vi "get ext error.vi"(5 "connection reference":T1, 6 "length":i32=1, 7 "sample data list":T2, 9 "seq std":dbl[][](array[numeric]), 10 "sample data":string[][](array[string]), 11 "unknown data in":dbl[][][](array[numeric])) -> (2 "normalized ratio":dbl[](array[numeric]), 3 "Array out":string[][](array[string]))   [LabVIEW 2016]
uses:
  <vilib>/addons/database/Connection.llb/Conn ObjectReference.ctl
  <vilib>/Analysis/baseanly.llb/Mean (DBL).vi
  <vilib>/addons/database/Connection.llb/Conn Execute.vi
  <vilib>/addons/database/Recordset.llb/Rec Fetch Recordset Data (R).vi
  <vilib>/addons/database/Recordset.llb/Rec Destroy - Connection.vi
  <vilib>/addons/database/NI_Database_API.lvlib
  <vilib>/Analysis/NI_AALBase.lvlib
panel:
  out "error out":errorcluster
  out "Array 2":string[][](array[string])
  out "unknown data in 4":dbl[][](array[numeric])
  out "subarray":dbl[](array[numeric])
  out "unknown data in 3":dbl[][](array[numeric])
  out "unknown data in 2":dbl[](array[numeric])
  out "Array":dbl[](array[numeric])
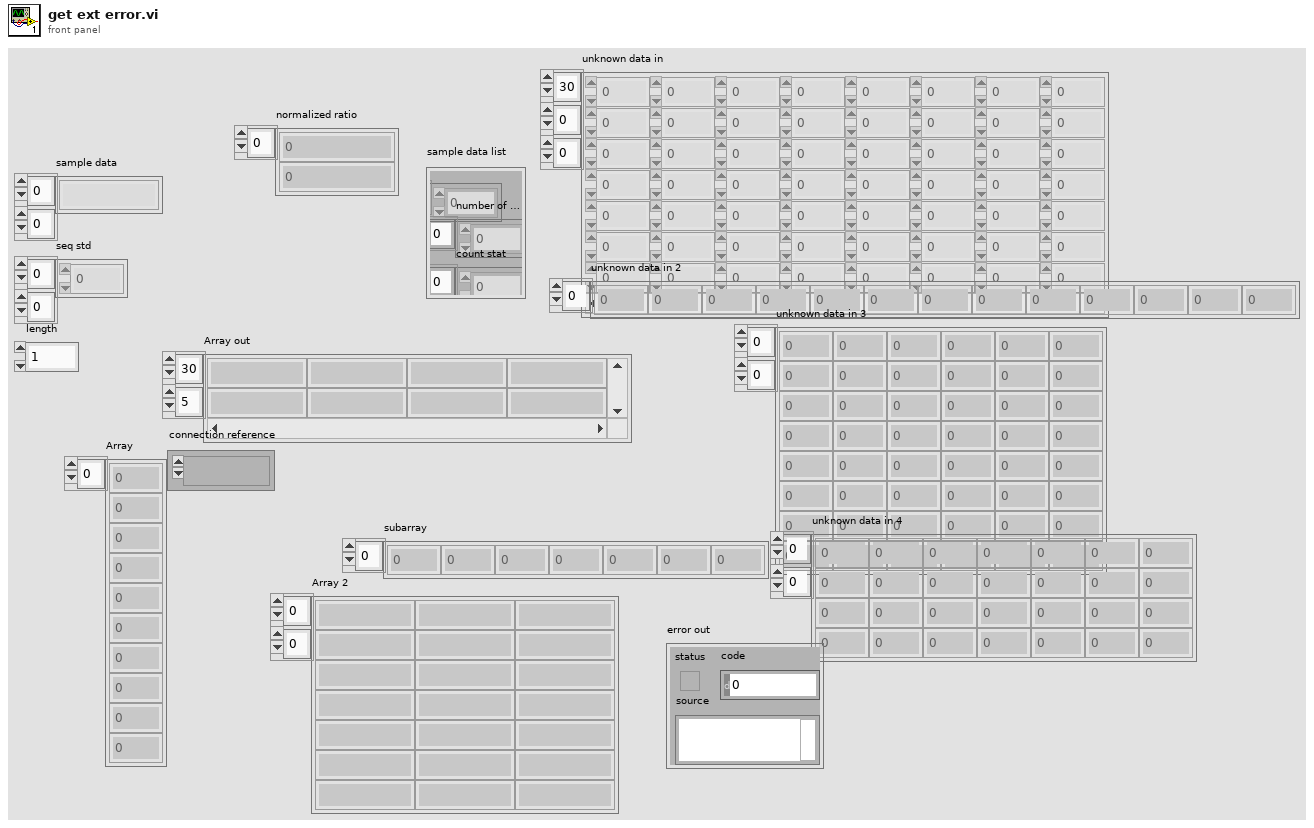
[diagram p1: front panel]
types:
  T1 = typedef "NI_Database_API.lvlib/Conn ObjectReference.ctl" = refnum<k1>
  T2 = cluster{"last currents":dbl[], "number of cycles":i32[], "count stat":dbl[]}
  T3 = typedef "NI_Database_API.lvlib/Rec ObjectReference.ctl" = refnum<k1>
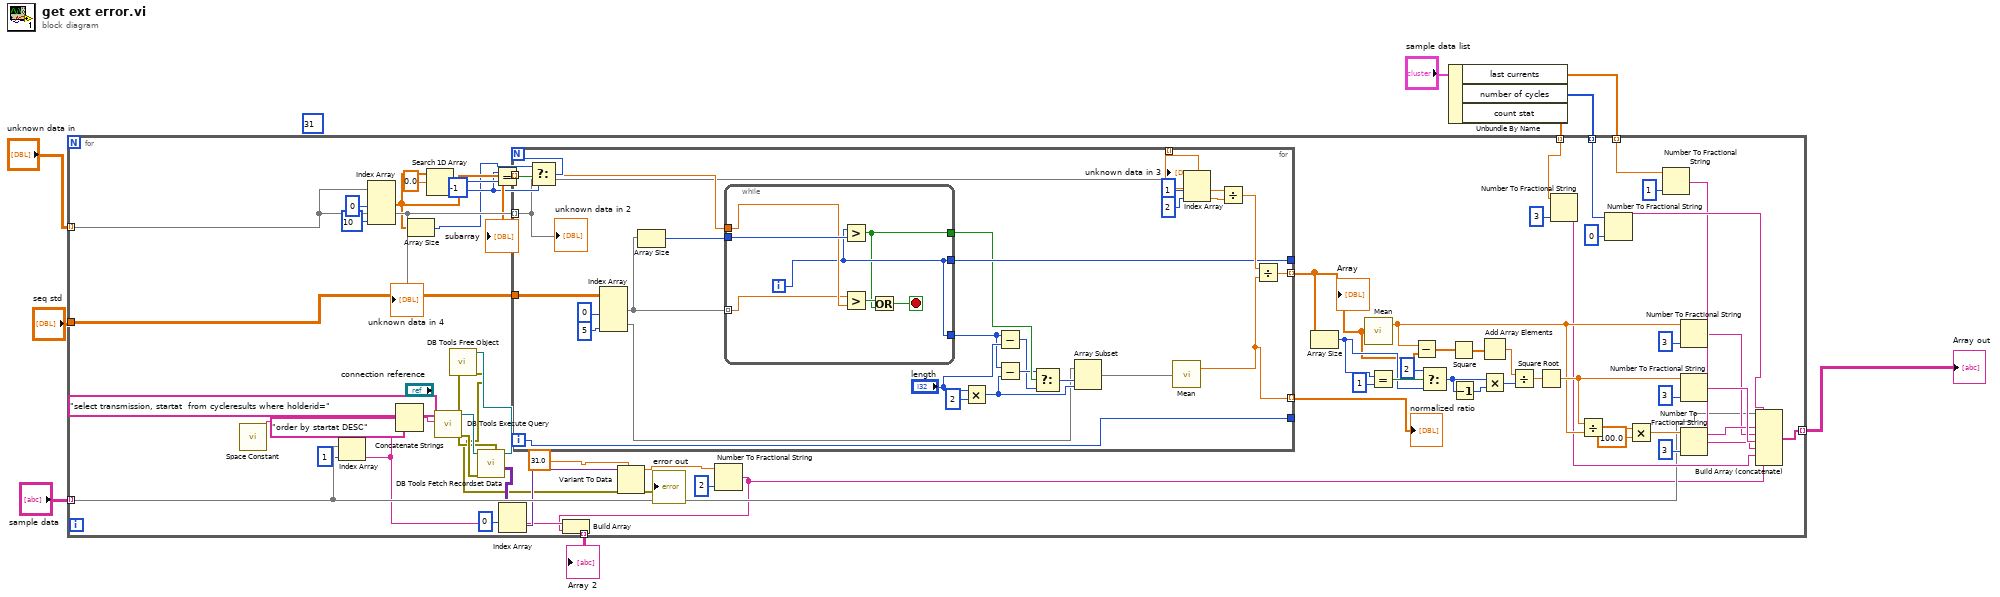
[diagram p0: block diagram]
diagram:
  (unwired) 31
  n1 = Unbundle By Name("sample data list") -> ("last currents"=w3:dbl[], "number of cycles"=w5:i32[], "count stat"=w4:dbl[])
  n2 = for {
    tunnel: "unknown data in" -> [w72] mode=indexing
    tunnel: "seq std" -> [w76]
    tunnel: "sample data" -> [w26] mode=indexing
    tunnel: [w74] -> w2 mode=indexing
    tunnel: w5 -> [w42] mode=indexing
    tunnel: w4 -> [w39] mode=indexing
    tunnel: w3 -> [w37] mode=indexing
    tunnel: [w18] -> w1 mode=indexing
    w22 = 0 ("disabled index (col)")
    n3 = call <vilib>:"Space Constant.vi"() -> ("String"=w24:string)
    n4 = Index Array(array=w26, index=1) -> (element=w19:string)
    n5 = Index Array(array=w72, index (col) #1=0 ("disabled index (col)"), index (col) #2=10 ("index (col)")) -> (element #1=w51:dbl[])  [unwired: 2 in, 1 out]
    "subarray" <- w51
    n6 = Concatenate Strings("select transmission, startat  from cycleresults where holderid=" ("string"), w19, w24, "order by startat DESC" ("string")) -> (w28:string)
    n7 = Array Size(array=w51) -> (size(s)=w44:i32)
    n8 = Search 1D Array(1D array=w51, element=0.0) -> (index of element=w48:i32)  [unwired: 1 in]
    n9 = call-poly <vilib>:"DB Tools Execute Query.vi"("SQL query"=w28, "connection reference"="connection reference") -> ("error out"=w30:errorcluster, "recordset reference"=w29:T3)  [unwired: 6 in]
    n10 = call-poly <vilib>:"DB Tools Fetch Recordset Data.vi"("error in (no error)"=w30, "recordset reference"=w29) -> ("error out"=w17:errorcluster, "recordset data"=w23:variant[][], "recordset reference out"=w15:T3)  [unwired: 3 in]
    n11 = call-poly <vilib>:"DB Tools Free Object.vi"("error in (no error)"=w17, "recordset reference"=w15) -> ("error out"=w14:errorcluster)  [unwired: 8 in, 1 out]
    n12 = Equal?(x=w48, y=-1) -> (x = y?=w49:bool)
    n13 = Index Array(array=w23, index (row)=w22, index (col)=w22) -> (element=w21:variant)
    n14 = Select(t=w44, s=w49, f=w48) -> (s? t:f=w33:i32)
    n15 = for {
      N: w33 -> [_]
      tunnel: w76 -> [w99]
      tunnel: w72 -> [w81] mode=indexing
      tunnel: w51 -> [w102] mode=indexing
      tunnel: [w91] -> w47 mode=indexing
      tunnel: [w90] -> _
      tunnel: [w83] -> w46 mode=indexing
      tunnel: [w82] -> _
      tunnel: [w81] -> w32 mode=indexing
      i -> [w82]
      n16 = Index Array(array=w99, index (col) #1=0 ("disabled index (col)"), index (col) #2=5 ("index (col)")) -> (element #1=w101:dbl[], element #2=w78:dbl[])  [unwired: 2 in]
      n17 = Array Size(array=w101) -> (size(s)=w100:i32)
      n18 = while {
        tunnel: w102 -> [w107]
        tunnel: w101 -> [w106] mode=indexing
        tunnel: w100 -> [w108]
        tunnel: [w105] -> w80
        tunnel: [w105] -> w90
        tunnel: [w104] -> w88
        i -> [w105]
        stop <- w109 stop-if-true
        n19 = Greater?(x=w105, y=w108) -> (0:w104:bool)
        n20 = Greater?(x=w106, y=w107) -> (0:w110:bool)
        n21 = Or(x=w110, y=w104) -> (x .or. y?=w109:bool)
      }
      n22 = Multiply(x="length", y=2) -> (x*y=w79:i32)
      n23 = Subtract(x=w80, y="length") -> (x-y=w84:i32)
      n24 = Subtract(x=w80, y=w79) -> (x-y=w86:i32)
      n25 = Select(t=w86, s=w88, f=w84) -> (s? t:f=w85:i32)
      n26 = Array Subset(array=w78, index=w85, length=w79) -> (w89:dbl[])
      n27 = call-poly <vilib>:"Mean.vi"("X"=w89) -> ("mean"=w83:dbl)  [unwired: 1 out]
      n28 = Index Array(array=w81, index #1=1 ("index"), index #2=2 ("index")) -> (element #1=w93:dbl, element #2=w94:dbl)
      n29 = Divide(x=w93, y=w94) -> (x/y=w92:dbl)
      n30 = Divide(x=w92, y=w83) -> (x/y=w91:dbl)
      "unknown data in 2" <- w81
    }
    "normalized ratio" <- w46
    "Array" <- w47
    "unknown data in 3" <- w32
    n31 = Variant To Data(error in=w14, type=31.0, Variant=w21) -> (data=w12:dbl, error out=→"error out":errorcluster)
    n32 = Number To Fractional String(number=w12, precision (6)=i16 2) -> (F-format string=w10:string)  [unwired: 2 in]
    n33 = Build Array(w19, w10) -> (w18:string[])
    n34 = Array Size(array=w47) -> (size(s)=w67:i32)
    n35 = call-poly <vilib>:"Mean.vi"("X"=w47) -> ("mean"=w61:dbl)  [unwired: 1 out]
    n36 = Equal?(x=w67, y=1) -> (x = y?=w69:bool)
    n37 = Subtract(x=w61, y=w47) -> (x-y=w71:dbl[])
    n38 = Select(t=2, s=w69, f=w67) -> (s? t:f=w59:i32)
    n39 = Square(x=w71) -> (x^2=w70:dbl[])
    n40 = Decrement(x=w59) -> (x-1=w58:i32)
    n41 = Add Array Elements(numeric array=w70) -> (sum=w65:dbl)
    n42 = Multiply(x=w59, y=w58) -> (x*y=w57:i32)
    n43 = Divide(x=w65, y=w57) -> (x/y=w64:dbl)
    n44 = Square Root(x=w64) -> (sqrt(x)=w62:dbl)
    n45 = Number To Fractional String(number=w39, precision (6)=i16 3) -> (F-format string=w36:string)  [unwired: 2 in]
    n46 = Divide(x=w62, y=w61) -> (x/y=w63:dbl)
    n47 = Number To Fractional String(number=w42, precision (6)=i16 0) -> (F-format string=w41:string)  [unwired: 2 in]
    n48 = Multiply(x=w63, y=100.0) -> (x*y=w53:dbl)
    n49 = Number To Fractional String(number=w37, precision (6)=i16 1) -> (F-format string=w35:string)  [unwired: 2 in]
    n50 = Number To Fractional String(number=w61, precision (6)=i16 3 ("width (-)")) -> (F-format string=w34:string)  [unwired: 2 in]
    n51 = Number To Fractional String(number=w62, precision (6)=i16 3 ("width (-)")) -> (F-format string=w55:string)  [unwired: 2 in]
    n52 = Number To Fractional String(number=w53, precision (6)=i16 3 ("width (-)")) -> (F-format string=w52:string)  [unwired: 2 in]
    n53 = Build Array (concatenate)(w26, w41, w35, w34, w55, w52, w36, w10) -> (w74:string[])
    "unknown data in 4" <- w72
  }
  "Array out" <- w2
  "Array 2" <- w1
